vi "myRIO_BRig_RT_dataMTrig_main__wWarmUp__v2.vi"(0 "input_dataMTrig":u16[](array[numeric]), 4 "input_Audio_trig_L":bool, 6 "input_WarmUp_2":bool) -> (14 "output_dataMTrig":u16[](array[numeric]), 16 "output_Solenoid_L":bool, 18 "output_Audio_L":bool)   [LabVIEW 2014]
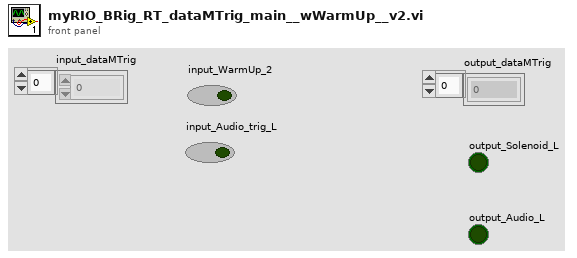
[diagram p1: front panel]
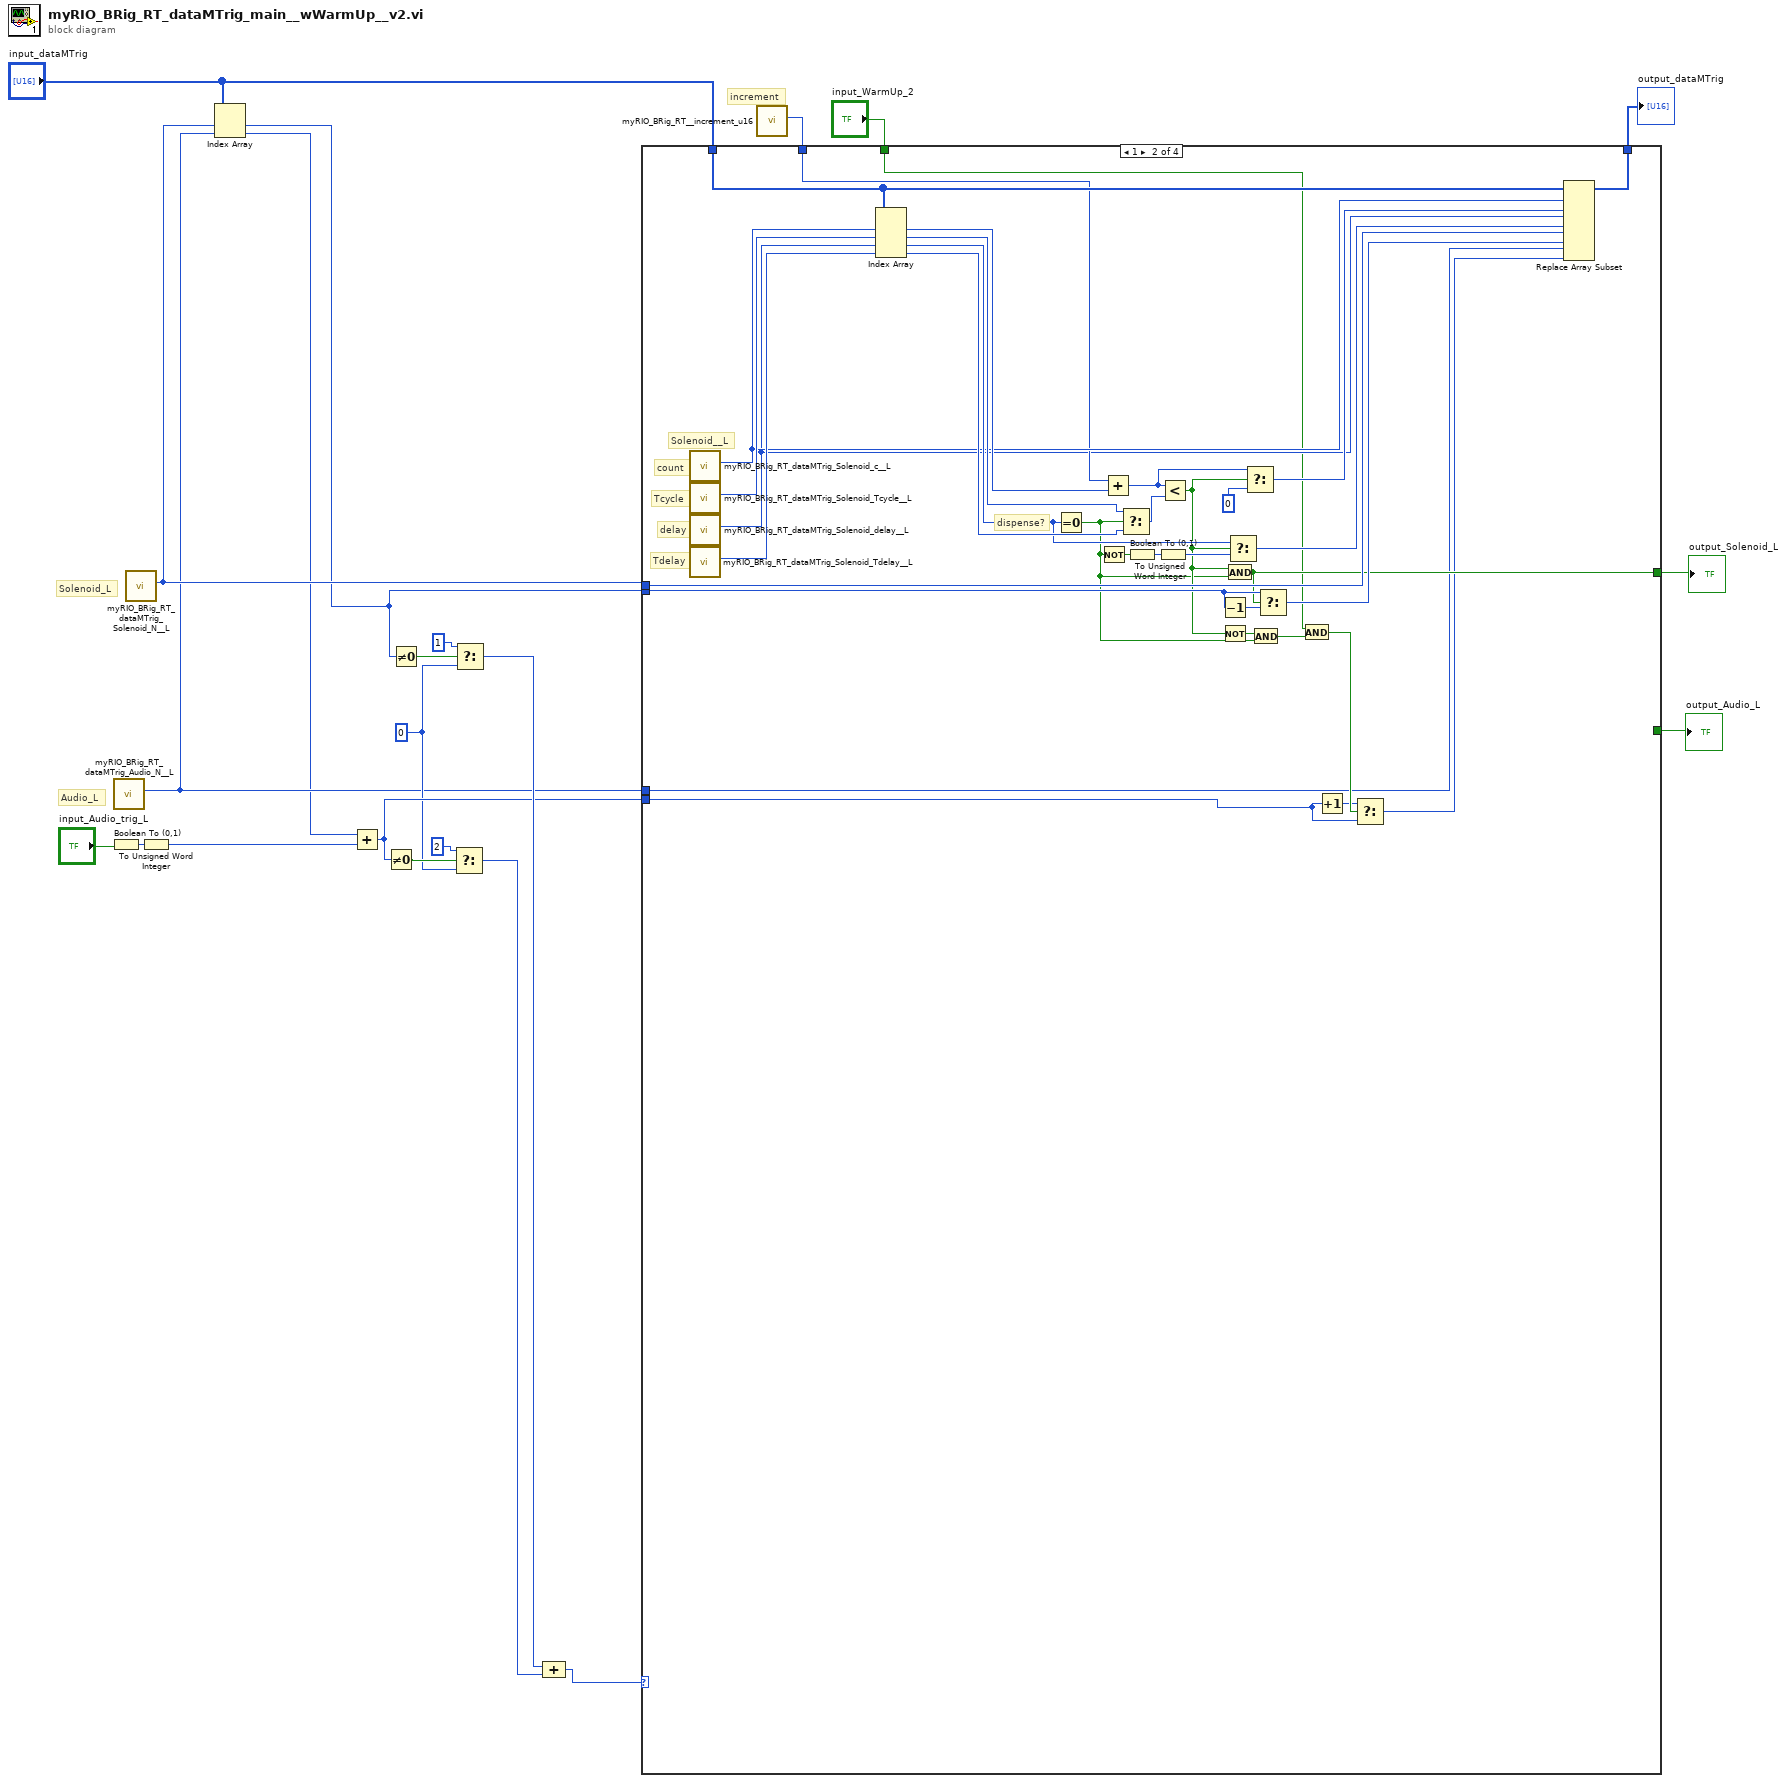
[diagram p0: block diagram]
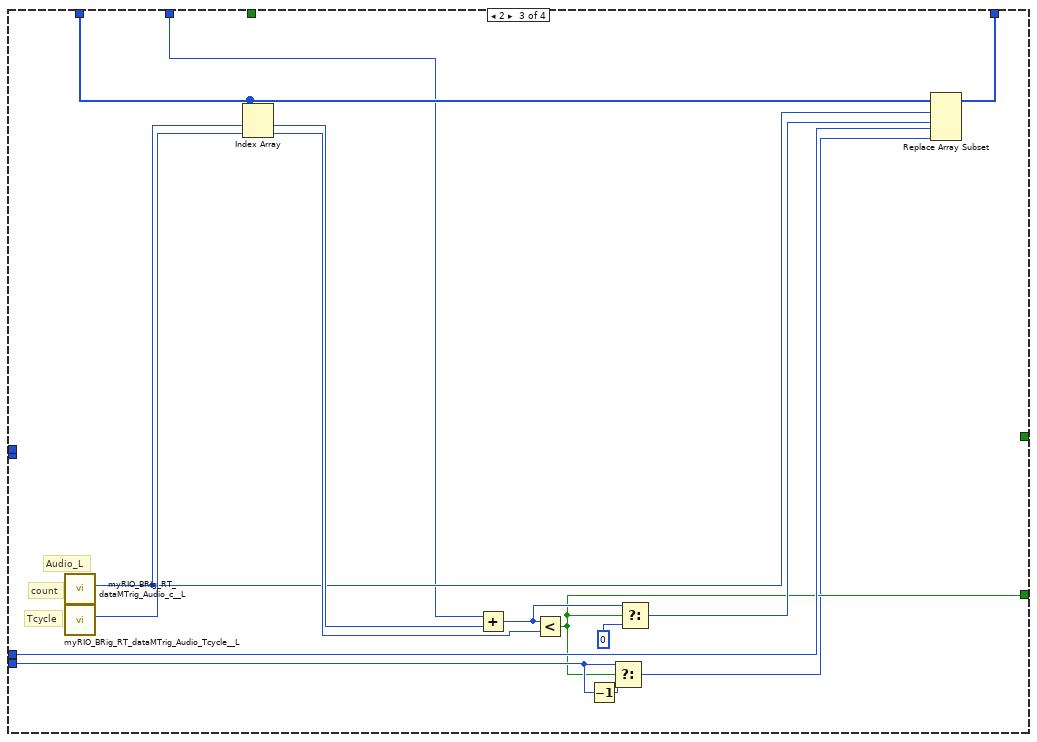
[diagram p3: hidden frame]
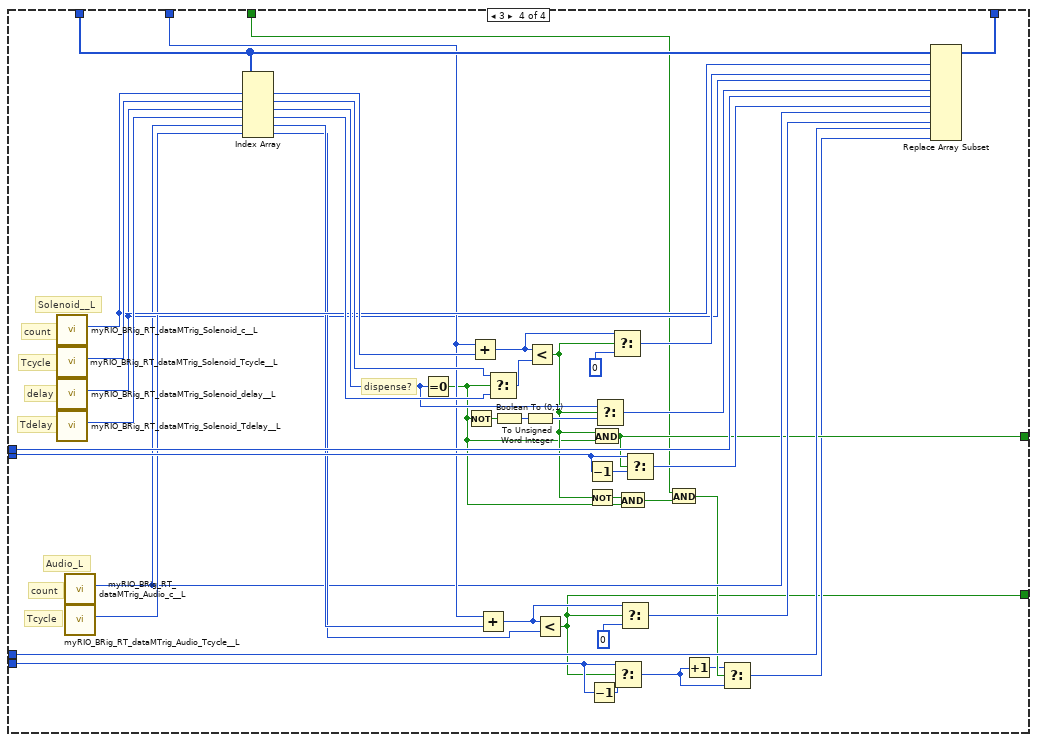
[diagram p4: hidden frame]
diagram:
  w5 = u8 0 ("f")
  # "increment"
  # "Audio_L"
  # "Solenoid_L"
  n1 = Boolean To (0,1)(Boolean="input_Audio_trig_L") -> (0, 1=w22:i16)
  n2 = call "myRIO_BRig_RT_dataMTrig_Audio_N__L.vi"() -> ("output_Audio_N__L"=w2:i32)  [unwired: 11 in]
  n3 = call "myRIO_BRig_RT_dataMTrig_Solenoid_N__L.vi"() -> ("output_Solenoid_N__L"=w13:i32)  [unwired: 11 in]
  n4 = To Unsigned Word Integer(number=w22) -> (unsigned 16bit integer=w21:u16)
  n5 = Index Array(array="input_dataMTrig", index #1=w13, index #2=w2) -> (element #1=w3:u16, element #2=w1:u16)
  n6 = Add(x=w1, y=w21) -> (x+y=w8:u16)
  n7 = Not Equal To 0?(x=w8) -> (x != 0?=w17:bool)
  n8 = Not Equal To 0?(x=w3) -> (x != 0?=w20:bool)
  n9 = Select(t=u8 2, s=w17, f=w5) -> (s? t:f=w4:u8)
  n10 = Select(t=u8 1, s=w20, f=w5) -> (s? t:f=w16:u8)
  n11 = Compound Arithmetic op=ADD(w16, w4) -> (w10:u8)
  n12 = call "myRIO_BRig_RT__increment_u16.vi"() -> ("output_increment__u16"=w14:u16)  [unwired: 11 in]
  n13 = case shown="1" w10 {
    tunnel: w3 -> [_ w57 _ w116]
    tunnel: "input_dataMTrig" -> [w23 w56 w72 w115]
    tunnel: w14 -> [_ w37 w58 w93]
    tunnel: w13 -> [_ w55 _ w114]
    tunnel: [w23 w54 w71 w113] -> w12
    tunnel: [_ w35 _ w84] -> w11
    tunnel: w2 -> [_ w25 w63 w87]
    tunnel: w8 -> [_ w26 w64 w88]
    tunnel: "input_WarmUp_2" -> [_ w28 _ w77]
    tunnel: [_ _ w60 w73] -> w6
    frame 0, Default {
    }
    frame 1 {
      # "dispense?"
      # "Tdelay"
      # "delay"
      # "Solenoid__L"
      # "Tcycle"
      # "count"
      n14 = call "myRIO_BRig_RT_dataMTrig_Solenoid_c__L.vi"() -> ("output_Solenoid_c__L"=w41:i32)  [unwired: 11 in]
      n15 = call "myRIO_BRig_RT_dataMTrig_Solenoid_Tcycle__L.vi"() -> ("output_Solenoid_Tcycle__L"=w49:i32)  [unwired: 11 in]
      n16 = call "myRIO_BRig_RT_dataMTrig_Solenoid_delay__L.vi"() -> ("output_Solenoid_delay__L"=w36:i32)  [unwired: 11 in]
      n17 = call "myRIO_BRig_RT_dataMTrig_Solenoid_Tdelay__L.vi"() -> ("output_Solenoid_Tdelay__L"=w48:i32)  [unwired: 11 in]
      n18 = Index Array(array=w56, index #1=w41, index #2=w49, index #3=w36, index #4=w48) -> (element #1=w53:u16, element #2=w47:u16, element #3=w44:u16, element #4=w46:u16)
      n19 = Equal To 0?(x=w44) -> (x = 0?=w31:bool)
      n20 = Not(x=w31) -> (.not. x?=w34:bool)
      n21 = Add(x=w37, y=w53) -> (x+y=w51:u16)
      n22 = Select(t=w47, s=w31, f=w46) -> (s? t:f=w45:u16)
      n23 = Boolean To (0,1)(Boolean=w34) -> (0, 1=w43:i16)
      n24 = To Unsigned Word Integer(number=w43) -> (unsigned 16bit integer=w42:u16)
      n25 = Less?(x=w51, y=w45) -> (x < y?=w33:bool)
      n26 = Decrement(x=w57) -> (x-1=w52:u16)
      n27 = Not(x=w33) -> (.not. x?=w32:bool)
      n28 = And(x=w33, y=w31) -> (x .and. y?=w35:bool)
      n29 = Select(t=w44, s=w33, f=w42) -> (s? t:f=w39:u16)
      n30 = Select(t=w51, s=w33, f=u16 0) -> (s? t:f=w40:u16)
      n31 = And(x=w32, y=w31) -> (x .and. y?=w30:bool)
      n32 = Select(t=w57, s=w35, f=w52) -> (s? t:f=w38:u16)
      n33 = And(x=w28, y=w30) -> (x .and. y?=w29:bool)
      n34 = Increment(x=w26) -> (x+1=w27:u16)
      n35 = Select(t=w27, s=w29, f=w26) -> (s? t:f=w24:u16)
      n36 = Replace Array Subset(array=w56, new element #1=w40, index #1=w41, new element #2=w39, index #2=w36, new element #3=w38, index #3=w55, new element #4=w24, index #4=w25) -> (w54:u16[])
    }
    frame 2 {
      # "Audio_L"
      # "Tcycle"
      # "count"
      n37 = call "myRIO_BRig_RT_dataMTrig_Audio_c__L.vi"() -> ("output_Audio_c__L"=w62:i32)  [unwired: 11 in]
      n38 = call "myRIO_BRig_RT_dataMTrig_Audio_Tcycle__L.vi"() -> ("output_Audio_Tcycle__L"=w70:i32)  [unwired: 11 in]
      n39 = Index Array(array=w72, index #1=w62, index #2=w70) -> (element #1=w67:u16, element #2=w66:u16)
      n40 = Add(x=w58, y=w67) -> (x+y=w69:u16)
      n41 = Less?(x=w69, y=w66) -> (x < y?=w60:bool)
      n42 = Decrement(x=w64) -> (x-1=w65:u16)
      n43 = Select(t=w64, s=w60, f=w65) -> (s? t:f=w59:u16)
      n44 = Select(t=w69, s=w60, f=u16 0) -> (s? t:f=w61:u16)
      n45 = Replace Array Subset(array=w72, new element #1=w61, index #1=w62, new element #2=w59, index #2=w63) -> (w71:u16[])
    }
    frame 3 {
      # "Audio_L"
      # "Tcycle"
      # "count"
      # "dispense?"
      # "Tdelay"
      # "delay"
      # "Solenoid__L"
      # "Tcycle"
      # "count"
      n46 = call "myRIO_BRig_RT_dataMTrig_Solenoid_c__L.vi"() -> ("output_Solenoid_c__L"=w100:i32)  [unwired: 11 in]
      n47 = call "myRIO_BRig_RT_dataMTrig_Solenoid_Tcycle__L.vi"() -> ("output_Solenoid_Tcycle__L"=w108:i32)  [unwired: 11 in]
      n48 = call "myRIO_BRig_RT_dataMTrig_Solenoid_delay__L.vi"() -> ("output_Solenoid_delay__L"=w89:i32)  [unwired: 11 in]
      n49 = call "myRIO_BRig_RT_dataMTrig_Solenoid_Tdelay__L.vi"() -> ("output_Solenoid_Tdelay__L"=w107:i32)  [unwired: 11 in]
      n50 = call "myRIO_BRig_RT_dataMTrig_Audio_c__L.vi"() -> ("output_Audio_c__L"=w86:i32)  [unwired: 11 in]
      n51 = call "myRIO_BRig_RT_dataMTrig_Audio_Tcycle__L.vi"() -> ("output_Audio_Tcycle__L"=w96:i32)  [unwired: 11 in]
      n52 = Index Array(array=w115, index #1=w100, index #2=w108, index #3=w89, index #4=w107, index #5=w86, index #6=w96) -> (element #1=w112:u16, element #2=w106:u16, element #3=w103:u16, element #4=w105:u16, element #5=w92:u16, element #6=w91:u16)
      n53 = Equal To 0?(x=w103) -> (x = 0?=w80:bool)
      n54 = Not(x=w80) -> (.not. x?=w83:bool)
      n55 = Add(x=w93, y=w112) -> (x+y=w110:u16)
      n56 = Add(x=w93, y=w92) -> (x+y=w95:u16)
      n57 = Select(t=w106, s=w80, f=w105) -> (s? t:f=w104:u16)
      n58 = Boolean To (0,1)(Boolean=w83) -> (0, 1=w102:i16)
      n59 = To Unsigned Word Integer(number=w102) -> (unsigned 16bit integer=w101:u16)
      n60 = Less?(x=w110, y=w104) -> (x < y?=w82:bool)
      n61 = Less?(x=w95, y=w91) -> (x < y?=w73:bool)
      n62 = Decrement(x=w116) -> (x-1=w111:u16)
      n63 = Not(x=w82) -> (.not. x?=w81:bool)
      n64 = Decrement(x=w88) -> (x-1=w90:u16)
      n65 = And(x=w82, y=w80) -> (x .and. y?=w84:bool)
      n66 = Select(t=w103, s=w82, f=w101) -> (s? t:f=w98:u16)
      n67 = Select(t=w110, s=w82, f=u16 0) -> (s? t:f=w99:u16)
      n68 = Select(t=w88, s=w73, f=w90) -> (s? t:f=w75:u16)
      n69 = And(x=w81, y=w80) -> (x .and. y?=w79:bool)
      n70 = Select(t=w95, s=w73, f=u16 0) -> (s? t:f=w85:u16)
      n71 = Select(t=w116, s=w84, f=w111) -> (s? t:f=w97:u16)
      n72 = And(x=w77, y=w79) -> (x .and. y?=w78:bool)
      n73 = Increment(x=w75) -> (x+1=w76:u16)
      n74 = Select(t=w76, s=w78, f=w75) -> (s? t:f=w74:u16)
      n75 = Replace Array Subset(array=w115, new element #1=w99, index #1=w100, new element #2=w98, index #2=w89, new element #3=w97, index #3=w114, new element #4=w85, index #4=w86, new element #5=w74, index #5=w87) -> (w113:u16[])
    }
  }
  "output_dataMTrig" <- w12
  "output_Solenoid_L" <- w11
  "output_Audio_L" <- w6
